vi "Add New Or Old Parameter.vi"(8 "old port?":bool, 9 "refresh listbox":T5[](array[typedef]), 10 "channel parameter":T1={"name"="", "direction"=enum."Rx", "default value"=0.0, "unit"="", "Parameter"={"start index"=0, "size"=1, "encoding"=enum."BNR", "signed"=FALSE, "scale multiplier"=1.0, "scale offset"=0.0}}) -> (1 "refresh listbox out":T5[](array[typedef]))   [LabVIEW 2020, in "Ballard ARINC 429 System Explorer.lvlib" / "Implementation.lvlib"]
uses:
  Types/Refresh Listbox.ctl
  Types/Refresh Symbols.ctl
  Shared/VS Channel Definition for Parameter.ctl
  Shared/Direction.ctl
  Shared/Parameter Definition.ctl
  Encoding and Decoding/Encoding.ctl
  Implementation.lvlib
  Encoding and Decoding/Encoding and Decoding.lvlib
panel:
  in  "OK":bool
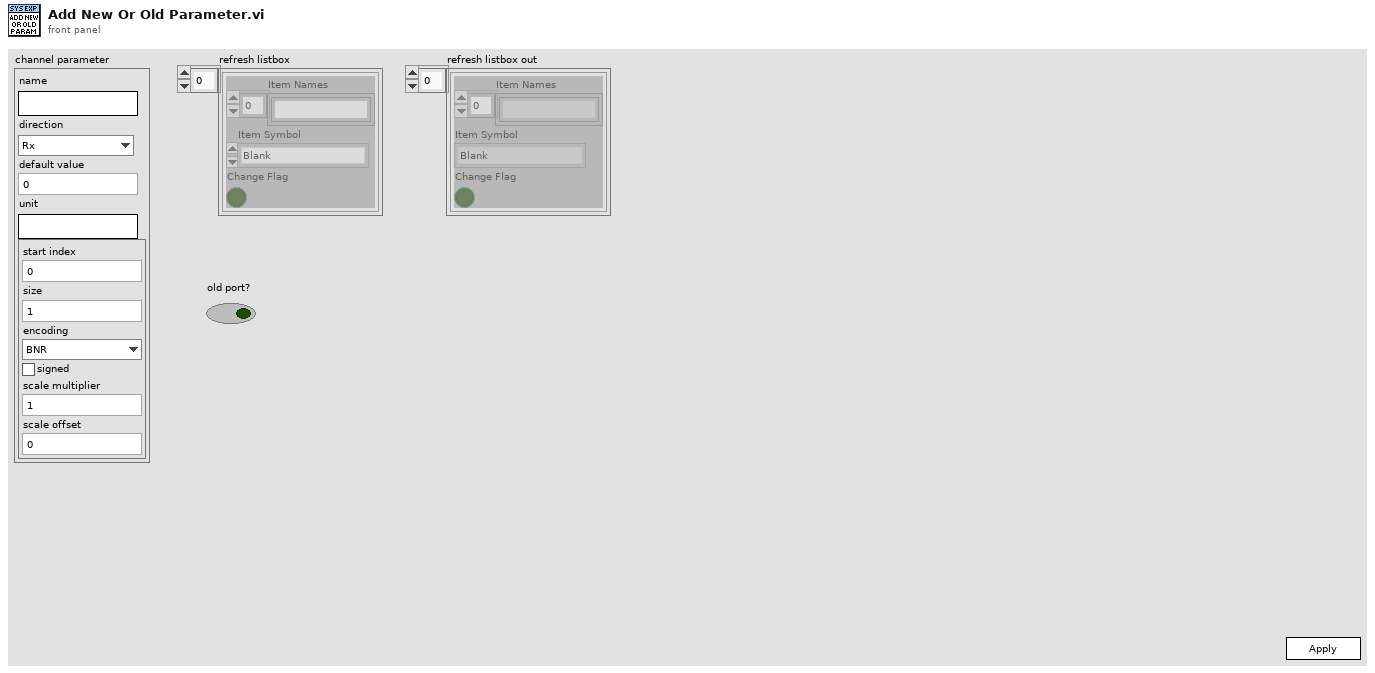
[diagram p1: front panel]
types:
  T1 = typedef "VS Channel Definition for Parameter.ctl" = cluster{"name":string, "direction":T2, "default value":dbl, "unit":string, "Parameter":T3}
  T2 = typedef "Direction.ctl" = enum16{"Rx", "Tx"}
  T3 = typedef "Parameter Definition.ctl" = cluster{"start index":i32, "size":i32, "encoding":T4, "signed":bool, "scale multiplier":dbl, "scale offset":dbl}
  T4 = typedef "Encoding and Decoding.lvlib/Encoding.ctl" = enum16{"BNR", "BCD", "Discrete"}
  T5 = typedef "Ballard ARINC 429 System Explorer.lvlib/Implementation.lvlib/Refresh Listbox.ctl" = cluster{"Item Names":string[], "Item Symbol":T6, "Change Flag":bool}
  T6 = typedef "Ballard ARINC 429 System Explorer.lvlib/Implementation.lvlib/Refresh Symbols.ctl" = enum16{"Blank", "Port", "Incoming", "Outgoing", "Label", "Word", "Parameter", "ARINC-429", "Config Files", "Channel Spec", "Item"}
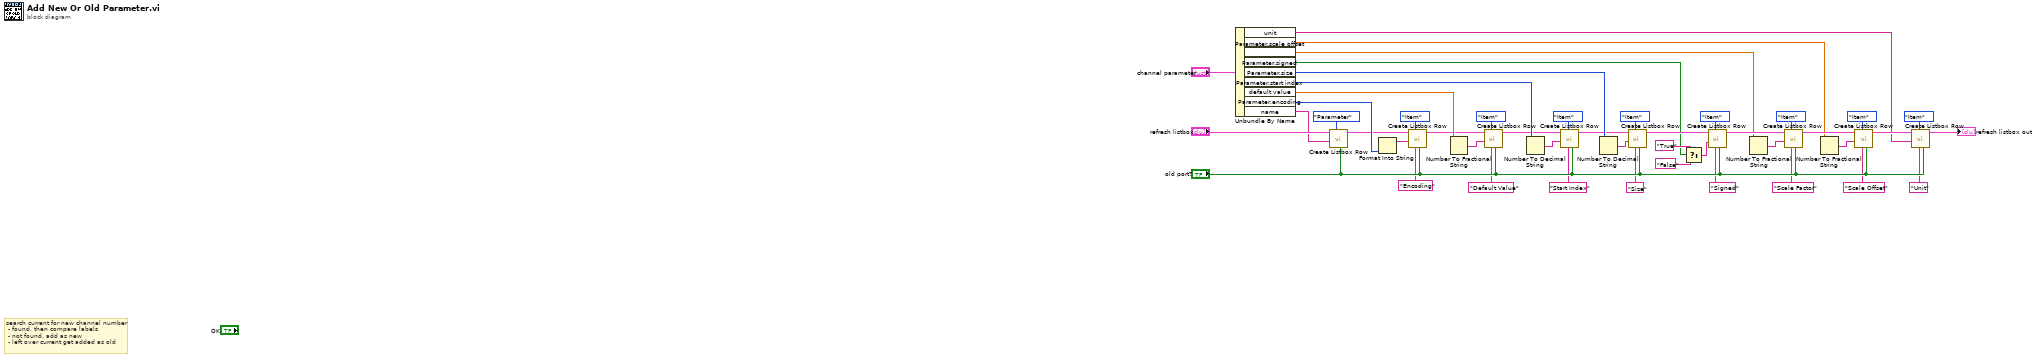
[diagram p0: block diagram]
diagram:
  # "search current for new channel number\n - found, then compare labels\n - not found, add as new\n - left over current get added as old"
  n1 = Unbundle By Name("channel parameter") -> ("unit"=w3:string, "Parameter.scale offset"=w6:dbl, "Parameter.scale multiplier"=w11:dbl, "Parameter.signed"=w16:bool, "Parameter.size"=w24:i32, "Parameter.start index"=w29:i32, "default value"=w34:dbl, "Parameter.encoding"=w40:T4, "name"=w43:string)
  n2 = call "Create Listbox Row.vi"("swap new and old (F)"="old port?", "refresh symbol (Blank)"=Refresh_Symbols."Parameter" ("Refresh Symbol (Blank)"), "new item"=w43, "refresh listbox"="refresh listbox") -> ("refresh listbox out"=w38:T5[])  [unwired: 7 in]
  n3 = Format Into String(w40) -> (resulting string=w41:string)  [unwired: 3 in, 1 out]
  n4 = call "Create Listbox Row.vi"("swap new and old (F)"="old port?", "override name"="Encoding" ("name"), "refresh symbol (Blank)"=Refresh_Symbols."Item" ("Refresh Symbol (Blank)"), "new item"=w41, "refresh listbox"=w38) -> ("refresh listbox out"=w33:T5[])  [unwired: 6 in]
  n5 = Number To Fractional String(number=w34) -> (F-format string=w35:string)  [unwired: 3 in]
  n6 = call "Create Listbox Row.vi"("swap new and old (F)"="old port?", "override name"="Default Value" ("name"), "refresh symbol (Blank)"=Refresh_Symbols."Item" ("Refresh Symbol (Blank)"), "new item"=w35, "refresh listbox"=w33) -> ("refresh listbox out"=w28:T5[])  [unwired: 6 in]
  n7 = Number To Decimal String(number=w29) -> (decimal integer string=w30:string)  [unwired: 1 in]
  n8 = call "Create Listbox Row.vi"("swap new and old (F)"="old port?", "override name"="Start Index" ("name"), "refresh symbol (Blank)"=Refresh_Symbols."Item" ("Refresh Symbol (Blank)"), "new item"=w30, "refresh listbox"=w28) -> ("refresh listbox out"=w23:T5[])  [unwired: 6 in]
  n9 = Number To Decimal String(number=w24) -> (decimal integer string=w27:string)  [unwired: 1 in]
  n10 = call "Create Listbox Row.vi"("swap new and old (F)"="old port?", "override name"="Size" ("name"), "refresh symbol (Blank)"=Refresh_Symbols."Item" ("Refresh Symbol (Blank)"), "new item"=w27, "refresh listbox"=w23) -> ("refresh listbox out"=w17:T5[])  [unwired: 6 in]
  n11 = Select(t="True", s=w16, f="False") -> (s? t:f=w20:string)
  n12 = call "Create Listbox Row.vi"("swap new and old (F)"="old port?", "override name"="Signed" ("name"), "refresh symbol (Blank)"=Refresh_Symbols."Item" ("Refresh Symbol (Blank)"), "new item"=w20, "refresh listbox"=w17) -> ("refresh listbox out"=w12:T5[])  [unwired: 6 in]
  n13 = Number To Fractional String(number=w11) -> (F-format string=w15:string)  [unwired: 3 in]
  n14 = call "Create Listbox Row.vi"("swap new and old (F)"="old port?", "override name"="Scale Factor" ("name"), "refresh symbol (Blank)"=Refresh_Symbols."Item" ("Refresh Symbol (Blank)"), "new item"=w15, "refresh listbox"=w12) -> ("refresh listbox out"=w7:T5[])  [unwired: 6 in]
  n15 = Number To Fractional String(number=w6) -> (F-format string=w8:string)  [unwired: 3 in]
  n16 = call "Create Listbox Row.vi"("swap new and old (F)"="old port?", "override name"="Scale Offset" ("name"), "refresh symbol (Blank)"=Refresh_Symbols."Item" ("Refresh Symbol (Blank)"), "new item"=w8, "refresh listbox"=w7) -> ("refresh listbox out"=w4:T5[])  [unwired: 6 in]
  n17 = call "Create Listbox Row.vi"("swap new and old (F)"="old port?", "override name"="Unit" ("name"), "refresh symbol (Blank)"=Refresh_Symbols."Item" ("Refresh Symbol (Blank)"), "new item"=w3, "refresh listbox"=w4) -> ("refresh listbox out"=→"refresh listbox out":T5[])  [unwired: 6 in]
